vi "3D_init.vi"() -> (2 "error out":errorcluster, 3 "reference out":refnum<vi>)   [LabVIEW 2012]
uses:
  <vilib>/picture/3D Picture Control/NI_3D Picture Control.lvlib
panel:
  in  "STL File Path":path
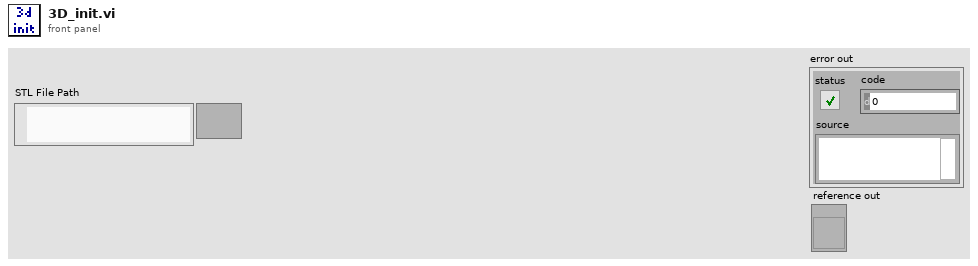
[diagram p1: front panel]
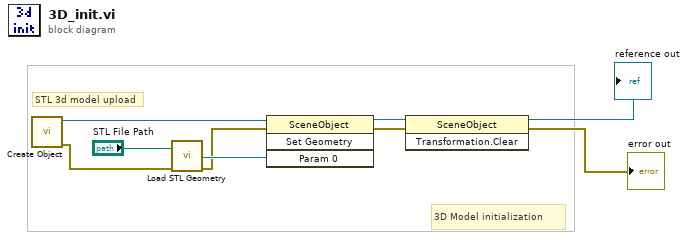
[diagram p0: block diagram]
diagram:
  # "3D Model initialization"
  # "STL 3d model upload"
  n1 = call <vilib>:"Create Object.vi"() -> ("error out"=w8:errorcluster, "Scene:New Object"=w6:refnum<vi>)  [unwired: 2 in, 8 out]
  n2 = call <vilib>:"Load STL Geometry.vi"("error in (no error)"=w8, "Model File"="STL File Path") -> ("error out"=w5:errorcluster, "New Mesh Refnum"=w7:refnum<vi>)  [unwired: 8 out]
  n3 = invoke class="SceneObject" method="Set Geometry"(reference=w6, error in=w5, "Param 0"=w7) -> (reference out=w4:refnum<vi>, error out=w3:errorcluster)  [unwired: 1 in, 2 out]
  n4 = invoke class="SceneObject" method="Transformation.Clear"(reference=w4, error in=w3) -> (reference out=→"reference out":refnum<vi>, error out=→"error out":errorcluster)  [unwired: 1 in, 1 out]
